vi "GetStreamingFilter.Do.vi"(8 "error in (no error)":errorcluster, 10 "State Variables":T3, 11 "gRPC Request":T1) -> (0 "error out":errorcluster, 2 "State Variables out":T3, 3 "gRPC Response":T14)   [LabVIEW 2025, in "bus_monitor_server_do.lvlib"]
uses:
  bus_monitor_server_do.lvlib
  Types/MainProcess.StateVariables.ctl
  Types/XNET.InitialSettings.ctl
  bus_monitor_server/RPC Messages/ni_bus_monitor_api_ConnectSettings.ctl
  bus_monitor_server/RPC Messages/ni_bus_monitor_api_CanMode.ctl
  bus_monitor_server/RPC Messages/ni_bus_monitor_api_Termination.ctl
  bus_monitor_server/RPC Messages/ni_bus_monitor_api_FdIsoMode.ctl
  bus_monitor_server/RPC Messages/ni_bus_monitor_api_FilterInfo.ctl
  bus_monitor_server/RPC Messages/ni_bus_monitor_api_DirectionFilter.ctl
  bus_monitor_server/RPC Messages/ni_bus_monitor_api_FrameFilter.ctl
  Types/StreamProcess.Refs.ctl
  Types/StreamProcess.VIRef.ctl
  bus_monitor_server/RPC Messages/ni_bus_monitor_api_Session.ctl
  bus_monitor_server/RPC Messages/ni_bus_monitor_api_GetStreamingFilterReply.ctl
  bus_monitor_server/RPC Messages/ni_bus_monitor_api_ErrorInfo.ctl
  bus_monitor_server/RPC Messages/ni_bus_monitor_api_GetStreamingFilterRequest.ctl
  bus_monitor_server/bus_monitor_server.lvlib
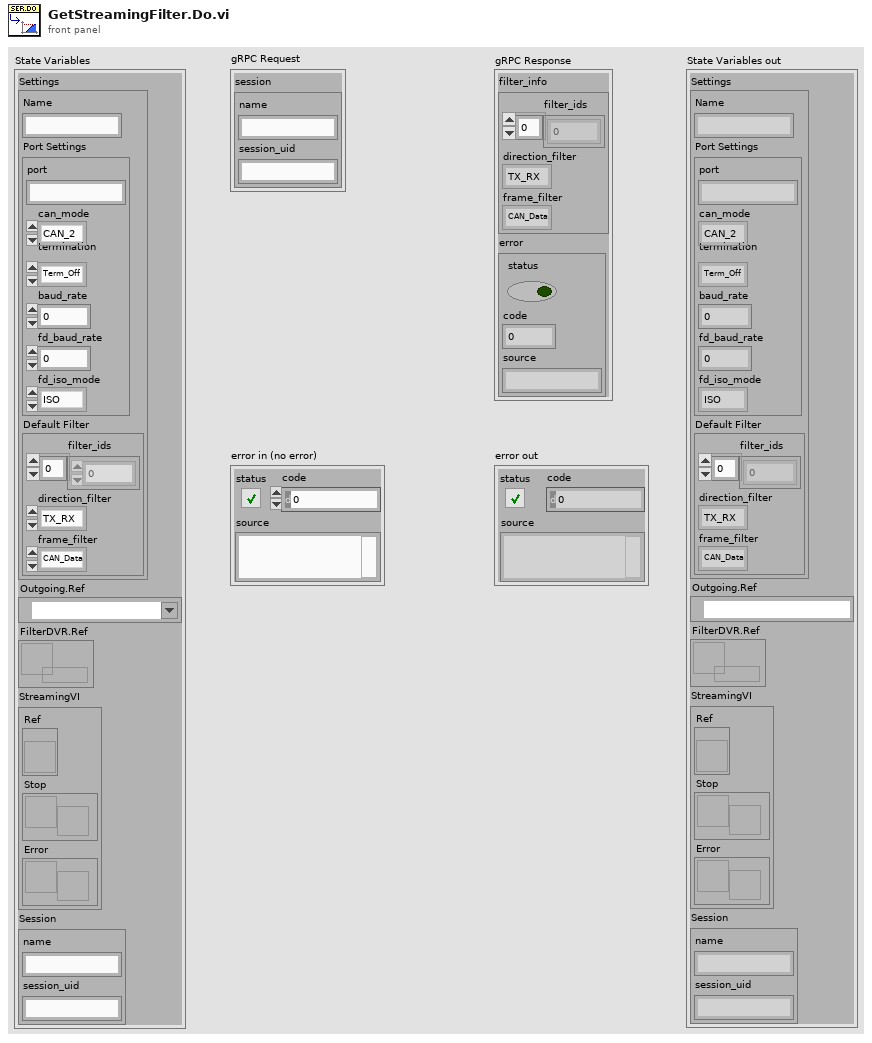
[diagram p1: front panel]
types:
  T1 = typedef "bus_monitor_server.lvlib/ni_bus_monitor_api_GetStreamingFilterRequest.ctl" = cluster{"session":T2}
  T2 = typedef "bus_monitor_server.lvlib/ni_bus_monitor_api_Session.ctl" = cluster{"name":string, "session_uid":string}
  T3 = typedef "bus_monitor_server_do.lvlib/MainProcess.StateVariables.ctl" = cluster{"Settings":T4, "Outgoing.Ref":refnum<k21>, "FilterDVR.Ref":refnum<data-value>, "StreamingVI":T12, "Session":T2}
  T4 = typedef "bus_monitor_server_do.lvlib/XNET.InitialSettings.ctl" = cluster{"Name":string, "Port Settings":T5, "Default Filter":T9}
  T5 = typedef "bus_monitor_server.lvlib/ni_bus_monitor_api_ConnectSettings.ctl" = cluster{"port":string, "can_mode":T6, "termination":T7, "baud_rate":u64, "fd_baud_rate":u64, "fd_iso_mode":T8}
  T6 = typedef "bus_monitor_server.lvlib/ni_bus_monitor_api_CanMode.ctl" = enum32{"CAN_2", "CAN_FD", "CAN_FD_BRS"}
  T7 = typedef "bus_monitor_server.lvlib/ni_bus_monitor_api_Termination.ctl" = enum32{"Term_Off", "Term_On"}
  T8 = typedef "bus_monitor_server.lvlib/ni_bus_monitor_api_FdIsoMode.ctl" = enum32{"ISO", "Non_ISO", "ISO_Legacy"}
  T9 = typedef "bus_monitor_server.lvlib/ni_bus_monitor_api_FilterInfo.ctl" = cluster{"filter_ids":u32[], "direction_filter":T10, "frame_filter":T11}
  T10 = typedef "bus_monitor_server.lvlib/ni_bus_monitor_api_DirectionFilter.ctl" = enum32{"TX_RX", "RX", "TX"}
  T11 = typedef "bus_monitor_server.lvlib/ni_bus_monitor_api_FrameFilter.ctl" = enum32{"CAN_Data", "CAN_Remote", "CAN_Bus_Error", "CAN_2_Data", "CAN_FD_Data", "CAN_FD_BRS_Data", "J1939_Data", "Delay", "Log_Trigger", "Start_Trigger", "All"}
  T12 = typedef "bus_monitor_server_do.lvlib/StreamProcess.Refs.ctl" = cluster{"Ref":T13, "Stop":refnum<notifier>, "Error":refnum<notifier>}
  T13 = typedef "bus_monitor_server_do.lvlib/StreamProcess.VIRef.ctl" = refnum<vi>
  T14 = typedef "bus_monitor_server.lvlib/ni_bus_monitor_api_GetStreamingFilterReply.ctl" = cluster{"filter_info":T9, "error":T15}
  T15 = typedef "bus_monitor_server.lvlib/ni_bus_monitor_api_ErrorInfo.ctl" = errorcluster
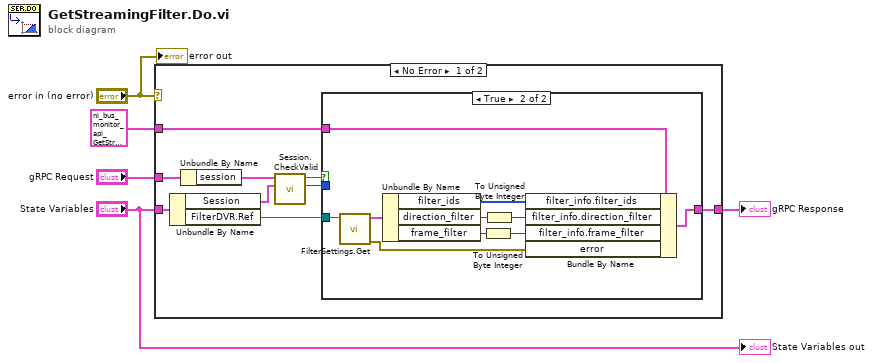
[diagram p0: block diagram]
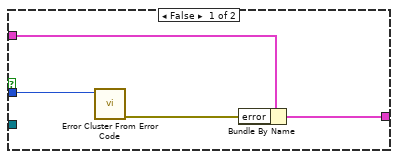
[diagram p2: hidden frame]
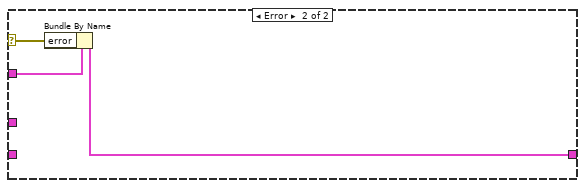
[diagram p3: hidden frame]
diagram:
  n1 = case shown="No Error" "error in (no error)" {
    selector: "error in (no error)" -> [_ w30]
    tunnel: "State Variables" -> [w14 _]
    tunnel: [w12 w29] -> w4
    tunnel: T14 {"filter_info"={"filter_ids"=[], "direction_filter"=enum."TX_RX", "frame_filter"=enum."CAN_Data"}, "error"={"status"=FALSE, "code"=0, "source"=""}} ("Message Data") -> [w11 w31]
    tunnel: "gRPC Request" -> [w10 _]
    frame No Error {
      n2 = Unbundle By Name(w14) -> ("Session"=w7:T2, "FilterDVR.Ref"=w13:refnum<data-value>)
      n3 = Unbundle By Name(w10) -> ("session"=w9:T2)
      n4 = call "Session.CheckValid.vi"("Cached Session"=w7, "requested session"=w9) -> ("Error Code"=w6:i32, "Valid?"=w8:bool)  [unwired: 8 in]
      n5 = case shown="True" w8 {
        tunnel: w13 -> [_ w21]
        tunnel: w11 -> [w18 w28]
        tunnel: [w17 w24] -> w12
        tunnel: w6 -> [w15 _]
        frame False {
          n6 = call <vilib>:"Error Cluster From Error Code.vi"("error code (0)"=w15) -> ("error out"=w16:errorcluster)  [unwired: 8 in]
          n7 = Bundle By Name(cluster=w18, "error"=w16) -> (w17:T14)
        }
        frame True {
          n8 = call "FilterSettings.Get.vi"("FilterDVR.Ref"=w21) -> ("error out"=w19:errorcluster, "Filter"=w20:T9)  [unwired: 9 in]
          n9 = Unbundle By Name(w20) -> ("filter_ids"=w27:u32[], "direction_filter"=w26:T10, "frame_filter"=w25:T11)
          n10 = To Unsigned Byte Integer(number=w25) -> (unsigned 8bit integer=w23:u8)
          n11 = To Unsigned Byte Integer(number=w26) -> (unsigned 8bit integer=w22:u8)
          n12 = Bundle By Name(cluster=w28, "filter_info.filter_ids"=w27, "filter_info.direction_filter"=w22, "filter_info.frame_filter"=w23, "error"=w19) -> (w24:T14)
        }
      }
    }
    frame Error {
      n13 = Bundle By Name(cluster=w31, "error"=w30) -> (w29:T14)
    }
  }
  "gRPC Response" <- w4
  "State Variables out" <- "State Variables"
  "error out" <- "error in (no error)"
